vi "plot_marginals.vi"() -> ()   [LabVIEW 2010]
uses:
  <vilib>/vision/NI_Vision_Development_Module.lvlib
panel:
  out "Y Marginal":sgl[](graph)
  out "X Marginal":sgl[](graph)
  in  "stop":bool
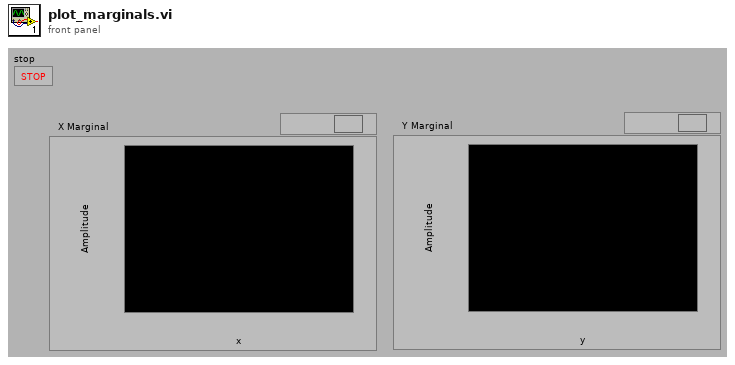
[diagram p1: front panel]
types:
  T1 = typedef "IMAQ Image.ctl" = refnum<image>
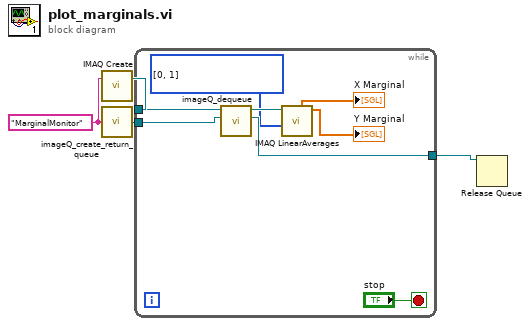
[diagram p0: block diagram]
diagram:
  w3 = "MarginalMonitor" ("Queue Name")
  n1 = call "IMAQ Create"("Image Name"=w3) -> ("New Image"=w2:T1)  [unwired: 4 in, 1 out]
  n2 = call "imageQ_create_return_queue.vi"("Queue Name"=w3) -> ("queue out"=w4:refnum<queue>)
  n3 = while {
    tunnel: w4 -> [w12]
    tunnel: w2 -> [w10]
    tunnel: [w8] -> w1
    stop <- "stop" stop-if-true
    w7 = i32[] [0, 1] items=["X Axis Averages", "Y Axis Averages", "X + Y Axis Averages", "X - Y Axis Averages"] ("Averages")
    n4 = call "imageQ_dequeue.vi"("Return queue"=w12, "Image Dst"=w10) -> ("Return queue out"=w8:refnum<queue>, "Image Dst Out"=w11:T1)  [unwired: 5 in, 3 out]
    n5 = call "IMAQ LinearAverages"("Averages"=w7, "Image Src"=w11) -> ("Y Axis Averages"=→"Y Marginal":sgl[], "X Axis Averages"=→"X Marginal":sgl[])  [unwired: 5 in, 3 out]
  }
  n6 = Release Queue(queue=w1) -> ()  [unwired: 2 in, 3 out]
